vi "Variant.BuildArrayFromElementArray.vi"(8 "error in (no error)":errorcluster, 9 "Dimensions":u32[](array[numeric]), 10 "Elements":variant[](array[variant]), 11 "Default Array":variant) -> (0 "error out":errorcluster, 3 "Output Array":variant)   [LabVIEW 2021, in "json.facade.lvlib"]
uses:
  json.facade.lvlib
  <vilib>/Utility/GetType.llb/Type Descriptor I16.ctl
  <vilib>/Utility/Data Type/NI_Data Type.lvlib
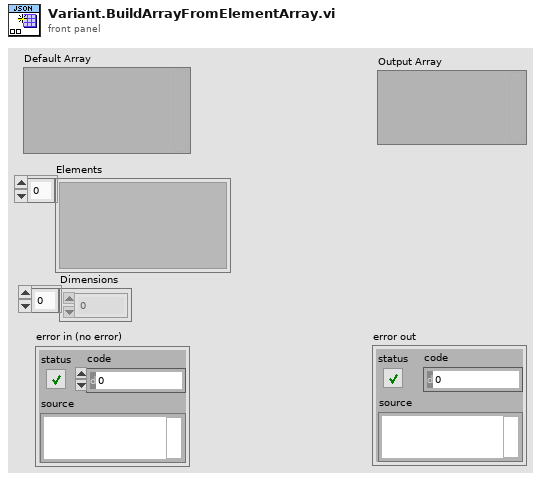
[diagram p1: front panel]
types:
  T1 = typedef "Type Descriptor I16.ctl" = i16
  T2 = typedef "NI_Data Type.lvlib/Data Type.ctl" = enum8{"Invalid Type", "Void", "I8", "I16", "I32", "I64", "U8", "U16", "U32", "U64", "Single Float", "Double Float", "Extended Float", "Single Complex", "Double Complex", "Extended Complex", "Enum U8", "Enum U16", "Enum U32", "Enum U64", "Single Float With Unit", "Double Float With Unit", "Extended Float With Unit", "Single Complex with Unit", "Double Complex with Unit", "Extended Complex with Unit", "Boolean", "String", "Path", "Picture", "Tag", "Array", "Cluster", "Variant", "LV Variant", "Waveform", "Timestamp", "Digital Waveform", "Digital Data", "ExpressData", "Refnum", "External Data", "VI", "Poly VI", "LabVIEW Class Instance", "Fixed Point", "Set Collection", "Map Collection"}
  T3 = typedef "Type Descriptor I16 Array.ctl" = T1[]
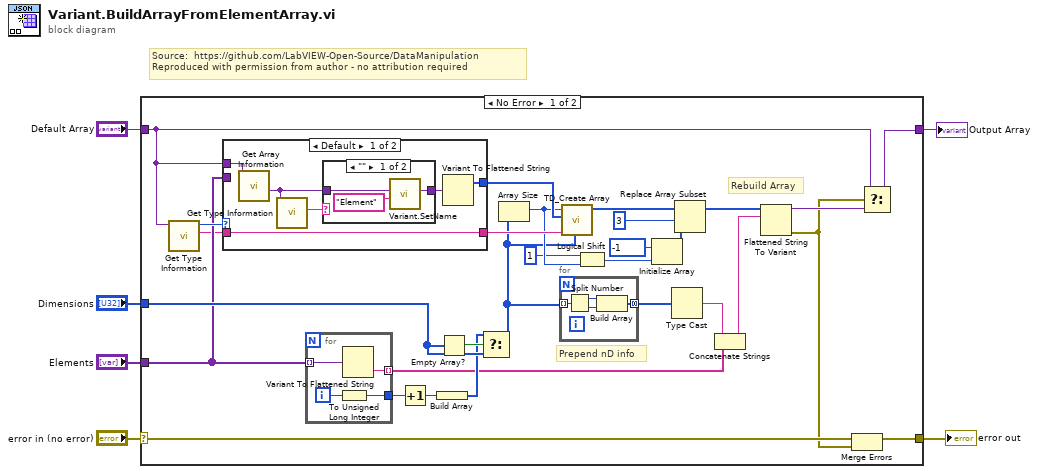
[diagram p0: block diagram]
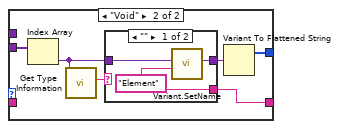
[diagram p3: hidden frame]
diagram:
  # "Source:  https://github.com/LabVIEW-Open-Source/DataManipulation\nReproduced with permission from author - no attribution required"
  n1 = case shown="No Error" "error in (no error)" {
    selector: "error in (no error)" -> [w32 w66]
    tunnel: "Dimensions" -> [w35 _]
    tunnel: "Elements" -> [w30 _]
    tunnel: [w33 w66] -> w4
    tunnel: [w34 w65] -> w3
    tunnel: "Default Array" -> [w29 w65]
    frame No Error {
      # "Prepend nD info"
      # "Rebuild Array"
      n2 = call <vilib>:"Get Type Information.vi"("variant"=w29) -> ("name"=w28:string, "type"=w31:T2)  [unwired: 6 in, 3 out]
      n3 = case shown="Default" w31 {
        tunnel: w30 -> [_ w51]
        tunnel: w29 -> [w41 _]
        tunnel: w28 -> [w36 _]
        tunnel: [w36 w46] -> w27
        tunnel: [w37 w47] -> w26
        frame Default {
          n4 = call <vilib>:"Get Array Information.vi"("variant"=w41) -> ("array element data type"=w38:variant)  [unwired: 7 in, 3 out]
          n5 = call <vilib>:"Get Type Information.vi"("variant"=w38) -> ("name"=w40:string)  [unwired: 6 in, 4 out]
          n6 = case shown="\"\"" w40 {
            tunnel: w38 -> [w44 w45]
            tunnel: [w43 w45] -> w39
            frame "" {
              n7 = call "Variant.SetName.vi"("Name"="Element" ("name"), "Variant"=w44) -> ("Named Variant"=w43:variant)  [unwired: 9 in]
            }
            frame Default {
            }
          }
          n8 = Variant To Flattened String(Variant=w39) -> (1:w37:i16[])  [unwired: 1 out]
        }
        frame "Void" {
          n9 = Index Array(array=w51) -> (element=w48:variant)  [unwired: 1 in]
          n10 = call <vilib>:"Get Type Information.vi"("variant"=w48) -> ("name"=w50:string)  [unwired: 6 in, 4 out]
          n11 = case shown="\"\"" w50 {
            selector: w50 -> [_ w55]
            tunnel: w48 -> [w54 w56]
            tunnel: [w53 w56] -> w49
            tunnel: [w52 w55] -> w46
            frame "" {
              w52 = "Element" ("name")
              n12 = call "Variant.SetName.vi"("Name"=w52, "Variant"=w54) -> ("Named Variant"=w53:variant)  [unwired: 9 in]
            }
            frame Default {
            }
          }
          n13 = Variant To Flattened String(Variant=w49) -> (1:w47:i16[])  [unwired: 1 out]
        }
      }
      n14 = for {
        tunnel: w30 -> [w60] mode=indexing
        tunnel: [w59] -> w8 mode=indexing
        tunnel: [w57] -> w12
        i -> [w58]
        n15 = To Unsigned Long Integer(number=w58) -> (unsigned 32bit integer=w57:u32)
        n16 = Variant To Flattened String(Variant=w60) -> (data string=w59:string)  [unwired: 1 out]
      }
      n17 = Increment(x=w12) -> (x+1=w11:u32)
      n18 = Build Array(w11) -> (w9:u32[])
      n19 = Empty Array?(array=w35) -> (empty?=w10:bool)
      n20 = Select(t=w9, s=w10, f=w35) -> (s? t:f=w7:u32[])
      n21 = Array Size(array=w7) -> (size(s)=w25:i32)
      n22 = for {
        tunnel: w7 -> [w64] mode=indexing
        tunnel: [w61] -> w20 mode=concatenating
        n23 = Split Number(x=w64) -> (hi(x)=w63:u16, lo(x)=w62:u16)
        n24 = Build Array(w63, w62) -> (w61:u16[])
      }
      n25 = call <vilib>:"TD_Create Array.vi"("Dim Lengths"=w7, "Name"=w27, "Array Elt"=w26, "N Dims"=w25) -> ("NewArray"=w16:T3)  [unwired: 7 in]
      n26 = Logical Shift(y=i16 1, x=w25) -> (x << y=w23:i32)
      n27 = Initialize Array(T1 -1 ("Numeric"), w23) -> (w19:T1[])
      n28 = Type Cast(x=w20) -> (*(type *) &x=w21:string)  [unwired: 1 in]
      n29 = Replace Array Subset(array=w16, new element=w19, index=3) -> (w17:T3)
      n30 = Concatenate Strings(w21, w8) -> (w24:string)
      n31 = Flattened String To Variant(6:w24, 7:w17) -> (0:w13:errorcluster, 3:w14:variant)  [unwired: 1 in]
      n32 = Merge Errors(w32, w13) -> (w33:errorcluster)
      n33 = Select(t=w29, s=w13, f=w14) -> (s? t:f=w34:variant)
    }
    frame Error {
    }
  }
  "error out" <- w4
  "Output Array" <- w3
